vi "VISA W.vi"(8 "errin":errorcluster, 11 "Chaîne":string) -> (0 "errout":errorcluster)   [LabVIEW 2020]
uses:
  VarGLO/Global PEAK.vi
panel:
  out "error out":errorcluster
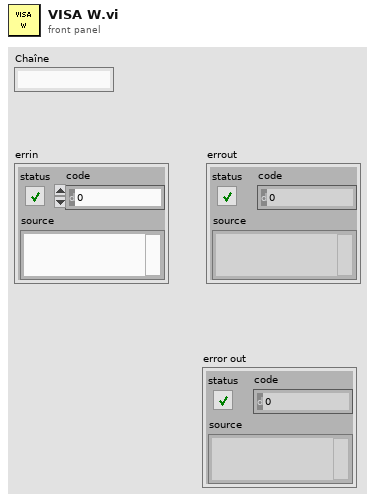
[diagram p1: front panel]
types:
  T1 = enum16{"open", "replace", "create", "open or create", "replace or create", "replace or create with confirmation"}
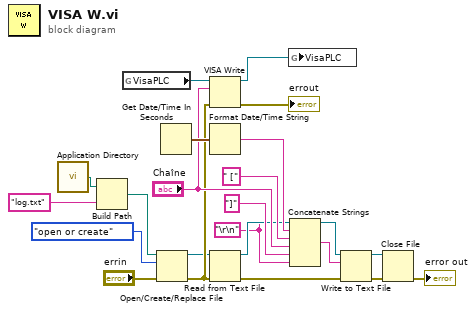
[diagram p0: block diagram]
diagram:
  w1 = "\r\n"
  n1 = call <vilib>:"Application Directory.vi"() -> ("Application Directory"=w18:path)
  n2 = Build Path ("Composer un chemin")(base path=w18, name or relative path="log.txt") -> (appended path=w17:path)
  n3 = global read "Global PEAK.vi" "VisaPLC"() -> (w21:refnum<visa-resource-name>)
  n4 = Open/Create/Replace File(file path (use dialog)=w17, error in="errin", operation (0:open)=T1."open or create") -> (refnum out=w4:refnum<file>, error out=w5:errorcluster)  [unwired: 3 in, 1 out]
  n5 = Get Date/Time In Seconds() -> (seconds since 1Jan1904=w11:timestamp)
  n6 = VISA Write(VISA resource name=w21, write buffer="Chaîne", error in (no error)=w5) -> (VISA resource name out=w22:refnum<visa-resource-name>, error out=→"errout":errorcluster)  [unwired: 1 out]
  n7 = Format Date/Time String(seconds (now)=w11) -> (date/time string=w10:string)  [unwired: 2 in]
  n8 = Read from Text File(file (use dialog)=w4, error in=w5) -> (refnum out=w3:refnum<file>, error out=w6:errorcluster)  [unwired: 2 in, 2 out]
  n9 = global write "Global PEAK.vi" "VisaPLC"(w22) -> ()
  n10 = Concatenate Strings(w1, w10, " [" ("string"), "Chaîne", "]" ("string"), w1) -> (w2:string)
  n11 = Write to Text File(file (use dialog)=w3, text=w2, error in=w6) -> (refnum out=w12:refnum<file>, error out=w14:errorcluster)  [unwired: 1 in, 1 out]
  n12 = Close File(refnum=w12, error in=w14) -> (error out=→"error out":errorcluster)  [unwired: 1 out]
